vi "Get Paths.vi"(10 "Assert Name":string, 11 "Path":path) -> (2 "Assert VI Path":path, 3 "Asserts Folder Path":path)   [LabVIEW 2016]
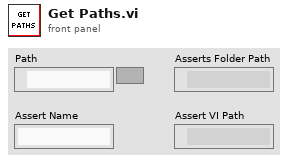
[diagram p1: front panel]
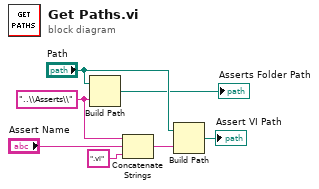
[diagram p0: block diagram]
diagram:
  w2 = "..\\Asserts\\" ("format string")
  n1 = Build Path(base path="Path", name or relative path=w2) -> (appended path=→"Asserts Folder Path":path)
  n2 = Concatenate Strings(w2, "Assert Name", ".vi" ("format string")) -> (w5:string)
  n3 = Build Path(base path="Path", name or relative path=w5) -> (appended path=→"Assert VI Path":path)
